vi "DownloadFileData.vi"(7 "Overwrite? (T)":bool=TRUE, 8 "error in (no error)":errorcluster, 9 "data":u8[](array[numeric]), 10 "Filename":string, 11 "VIA in":refnum<class "VIA.lvclass">) -> (0 "error out":errorcluster, 1 "bytes written":u32, 2 "Filename on NXT\\EV3":string, 3 "VIA out":refnum<class "VIA.lvclass">)   [LabVIEW 2012, in "VIA.lvclass"]
uses:
  <vilib>/NXT/LegoClasses/VIA/VIA.lvclass
  <vilib>/Utility/error.llb/DialogType.ctl
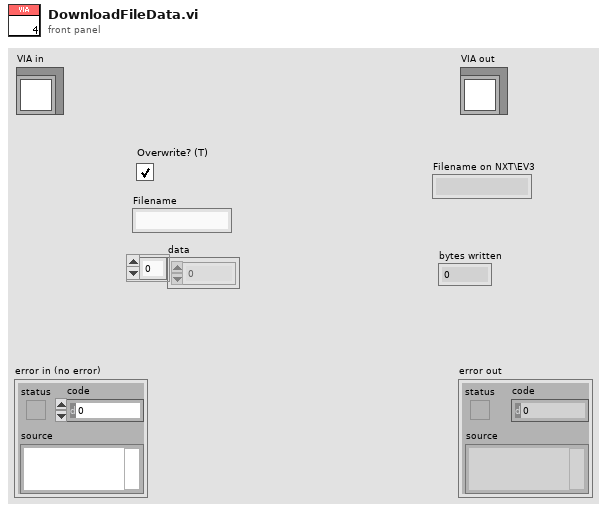
[diagram p1: front panel]
types:
  T1 = enum16{"open", "replace", "create", "open or create", "replace or create", "replace or create with confirmation"}
  T2 = typedef "DialogType.ctl" = u16
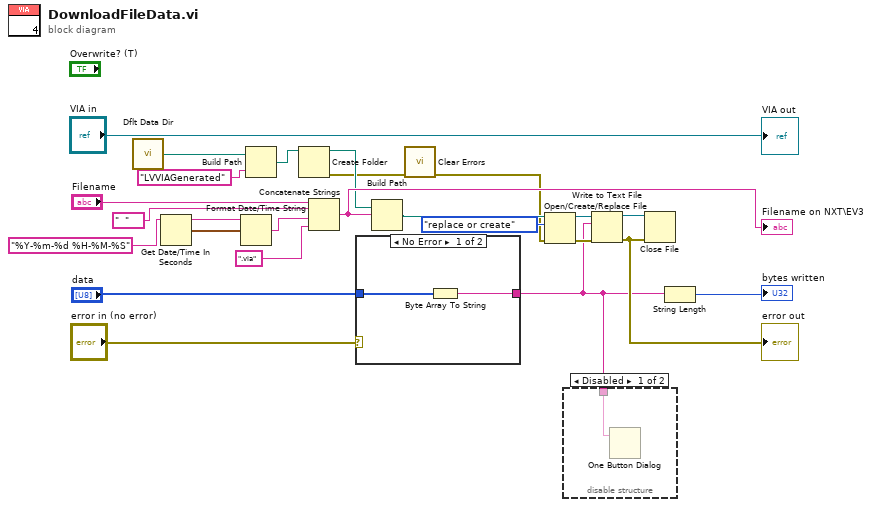
[diagram p0: block diagram]
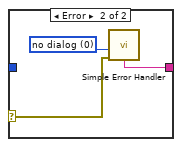
[diagram p3: hidden frame]
diagram:
  n1 = call <vilib>:"Dflt Data Dir.vi"() -> ("App:Default Data Directory"=w9:path)
  n2 = Get Date/Time In Seconds() -> (seconds since 1Jan1904=w11:timestamp)
  n3 = Format Date/Time String(time format string (%c)="%Y-%m-%d %H-%M-%S", seconds (now)=w11) -> (date/time string=w12:string)  [unwired: 1 in]
  n4 = Build Path(base path=w9, name or relative path="LVVIAGenerated" ("file (use dialog)")) -> (appended path=w7:path)
  n5 = Create Folder(path (use dialog)=w7) -> (created path=w6:path, error out=w5:errorcluster)  [unwired: 2 in, 1 out]
  n6 = Concatenate Strings("Filename", "  " ("string"), w12, ".via" ("string")) -> (w20:string)
  "Filename on NXT\\EV3" <- w20
  n7 = case shown="No Error" "error in (no error)" {
    selector: "error in (no error)" -> [_ w29]
    tunnel: "data" -> [w26 _]
    tunnel: [w25 w27] -> w1
    frame No Error {
      n8 = Byte Array To String(unsigned byte array=w26) -> (string=w25:string)
    }
    frame Error {
      w28 = T2 0 items=["no dialog", "OK message", "continue or stop message", "OK message + warnings", "continue/stop + warnings"] ("type of dialog (OK msg:1)")
      n9 = call <vilib>:"Simple Error Handler.vi"("type of dialog (OK msg:1)"=w28, "error in (no error)"=w29) -> ("message"=w27:string)  [unwired: 3 in, 4 out]
    }
  }
  n10 = Build Path(base path=w6, name or relative path=w20) -> (appended path=w16:path)
  n11 = call <vilib>:"Clear Errors.vi"("error in (no error)"=w5) -> ("error out"=w4:errorcluster)  [unwired: 6 in]
  n12 = Open/Create/Replace File(file path (use dialog)=w16, error in=w4, operation (0:open)=T1."replace or create") -> (refnum out=w15:refnum<file>, error out=w13:errorcluster)  [unwired: 3 in, 1 out]
  n13 = disable-structure shown="Disabled" {
    disable-tunnel: w1 -> [w30 _]
    frame Disabled {
      n14 = One Button Dialog(message=w30) -> ()  [unwired: 1 in, 1 out]
    }
    frame Enabled {
    }
  }
  n15 = Write to Text File(file (use dialog)=w15, text=w1, error in=w13) -> (refnum out=w2:refnum<file>, error out=w3:errorcluster)  [unwired: 1 in, 1 out]
  "error out" <- w3
  n16 = Close File(refnum=w2, error in=w3) -> ()  [unwired: 2 out]
  n17 = String Length(string=w1) -> (length=→"bytes written":i32)
  "VIA out" <- "VIA in"
